vi "CLUSTER JOYSTICK VALUES.vi"(9 "Axes":dbl[][](array[numeric]), 10 "Buttons":bool[][](array[boolean]), 11 "POVs":i16[][](array[numeric])) -> (2 "Joystick values":T1(array[cluster]))   [LabVIEW 2020]
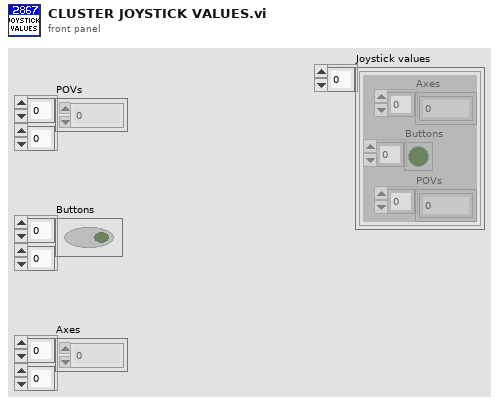
[diagram p1: front panel]
types:
  T1 = cluster{"Axes":dbl[], "Buttons":bool[], "POVs":i16[]}[]
  T2 = cluster{"Axes":dbl[], "Buttons":bool[], "POVs":i16[]}
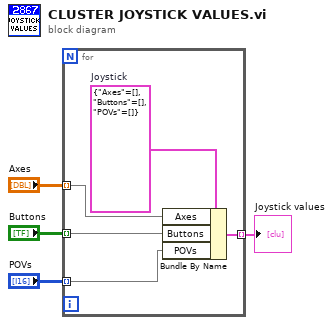
[diagram p0: block diagram]
diagram:
  n1 = for {
    tunnel: "Axes" -> [w8] mode=indexing
    tunnel: "Buttons" -> [w7] mode=indexing
    tunnel: "POVs" -> [w6] mode=indexing
    tunnel: [w5] -> w1 mode=indexing
    w9 = T2 {"Axes"=[], "Buttons"=[], "POVs"=[]}  # Joystick
    n2 = Bundle By Name(cluster=w9, "Axes"=w8, "Buttons"=w7, "POVs"=w6) -> (w5:T2)
  }
  "Joystick values" <- w1
